vi "Analyze.vi"(8 "error in (no error)":errorcluster, 10 "Image in":T1, 11 "Analyze Fluence in":refnum<class "Analyze Fluence.lvclass">) -> (0 "error out":errorcluster, 1 "Result":refnum<class "Analyze Results Base.lvclass">, 2 "Image out":T1, 3 "Analyze Fluence out":refnum<class "Analyze Fluence.lvclass">)   [LabVIEW 2014, in "Analyze.lvlib" / "Analyze Fluence.lvclass"]
doc: "In Variant Attributes to provide:\nEnergy: Energy in J\nROI: Image Display ROI Deskriptor\n\nOut Variant Attributes:\nFluence Infos: Array of Fluence Info.ctl\nMax Fluence: Maximal detected Fluence in J/cm^2"
uses:
  Analyze Fluence.lvclass
  <vilib>/vision/Image Controls.llb/IMAQ Image.ctl
  Results and Overlays/Results Base/Analyze Results Base.lvclass
  Results and Overlays/Results Fluence/Analyze Results Fluence.lvclass
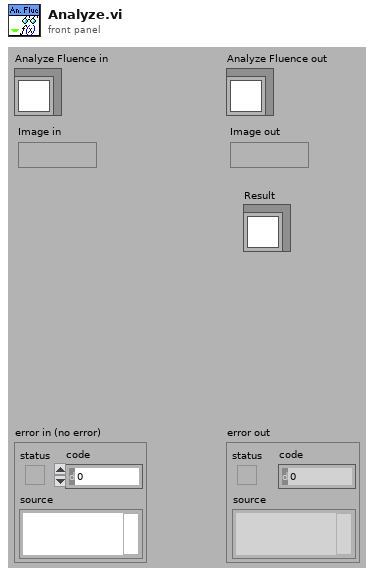
[diagram p1: front panel]
types:
  T1 = typedef "IMAQ Image.ctl" = refnum<image>
  T2 = typedef "Analyze.lvlib/Analyze Fluence.lvclass/Fluence Info.ctl" = cluster{"Fluence J/cm^2":dbl[unit], "Energy in Area":dbl[unit], "max value":i64, "Max fluence area":cluster{"Left":i32, "Top":i32, "Right":i32, "Bottom":i32}}
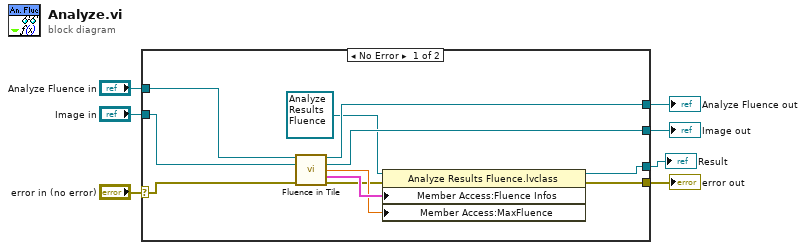
[diagram p0: block diagram]
diagram:
  n1 = case shown="No Error" "error in (no error)" {
    selector: "error in (no error)" -> [w9 w20]
    tunnel: [w18 w19] -> w7
    tunnel: [w11 w20] -> w6
    tunnel: "Analyze Fluence in" -> [w17 w19]
    tunnel: "Image in" -> [w10 w21]
    tunnel: [w16 w21] -> w3
    tunnel: [w8 _] -> w1
    frame No Error {
      n2 = call "Fluence in Tile.vi"("Analyze Fluence in"=w17, "Image in"=w10, "error in (no error)"=w9) -> ("Analyze Fluence out"=w18:refnum<class "Analyze Fluence.lvclass">, "Image Dst Out"=w16:T1, "Max Fluence"=w13:dbl[unit], "fluence infos"=w14:T2[], "error out"=w12:errorcluster)  [unwired: 8 in]
      n3 = property class="Analyze Results Fluence.lvclass"(reference=refnum<class "Analyze Results Fluence.lvclass"> refnum ("Analyze Results Fluence.lvclass"), error in=w12, "Member Access:Fluence Infos"=w14, "Member Access:MaxFluence"=w13) -> (reference out=w8:refnum<class "Analyze Results Fluence.lvclass">, error out=w11:errorcluster)
    }
    frame Error {
    }
  }
  "error out" <- w6
  "Analyze Fluence out" <- w7
  "Image out" <- w3
  "Result" <- w1
